vi "WaveformComponent, Append Dead Time.vi"(0 "waveform in":waveform(dbl)={"t0"=timestamp(3474820848.0780005 s since 1904-01-01), "dt"=nan, "Y"=[]}, 1 "frequency":dbl[unit]=nan format="%.1f", 2 "level (0.0)":dbl[unit] format="%.3f") -> (3 "waveform out":waveform(dbl)={"t0"=timestamp(-9593225999.921999 s since 1904-01-01), "dt"=nan, "Y"=[]})   [LabVIEW 2010]
uses:
  <vilib>/Waveform/WDTOps.llb/WDT Waveform Duration DBL.vi
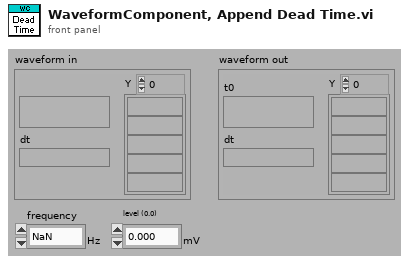
[diagram p1: front panel]
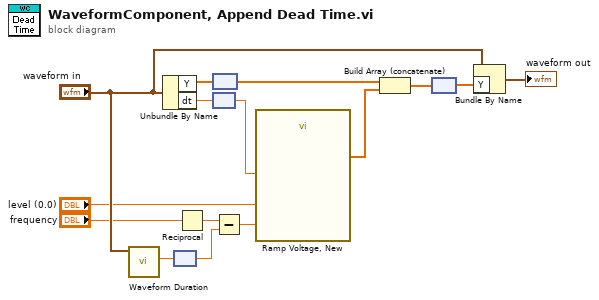
[diagram p0: block diagram]
diagram:
  n1 = call-poly <vilib>:"Waveform Duration.vi"("waveform in"="waveform in") -> ("duration"=w4:dbl)  [unwired: 8 in, 2 out]
  n2 = Unbundle By Name("waveform in") -> ("Y"=w13:dbl[], "dt"=w12:dbl)
  n3 = node(w4) -> (w3:dbl[unit])
  n4 = Reciprocal(x="frequency") -> (1/x=w5:dbl[unit])
  n5 = node(w13) -> (w10:dbl[unit][])
  n6 = node(w12) -> (w11:dbl[unit])
  n7 = Subtract(x=w5, y=w3) -> (x-y=w2:dbl[unit])
  n8 = call "Ramp Voltage, New.vi"("offset (0.0)"="level (0.0)", "dt"=w11, "total time"=w2) -> ("ramp"=w14:dbl[unit][])  [unwired: 2 in]
  n9 = Build Array (concatenate)(w10, w14) -> (w9:dbl[unit][])
  n10 = node(w9) -> (w15:dbl[])
  n11 = Bundle By Name(cluster="waveform in", "Y"=w15) -> (→"waveform out":waveform(dbl))
